vi "idontcare2.vi"() -> ()   [LabVIEW 2013]
panel:
  out "2D Picture":picture
  in  "Send Button":bool
  in  "GAIN2":dbl
  in  "GAIN1":dbl
  out "Rec Extra 4 Angle":dbl=2.8
  out "Rec Extra 3 Velocity":dbl=2.9
  out "Y":dbl=11.0
  out "X":dbl=3.0
  in  "Size of Rectangle":dbl=25.0
  in  "Display History":bool=TRUE
  in  "stop":bool
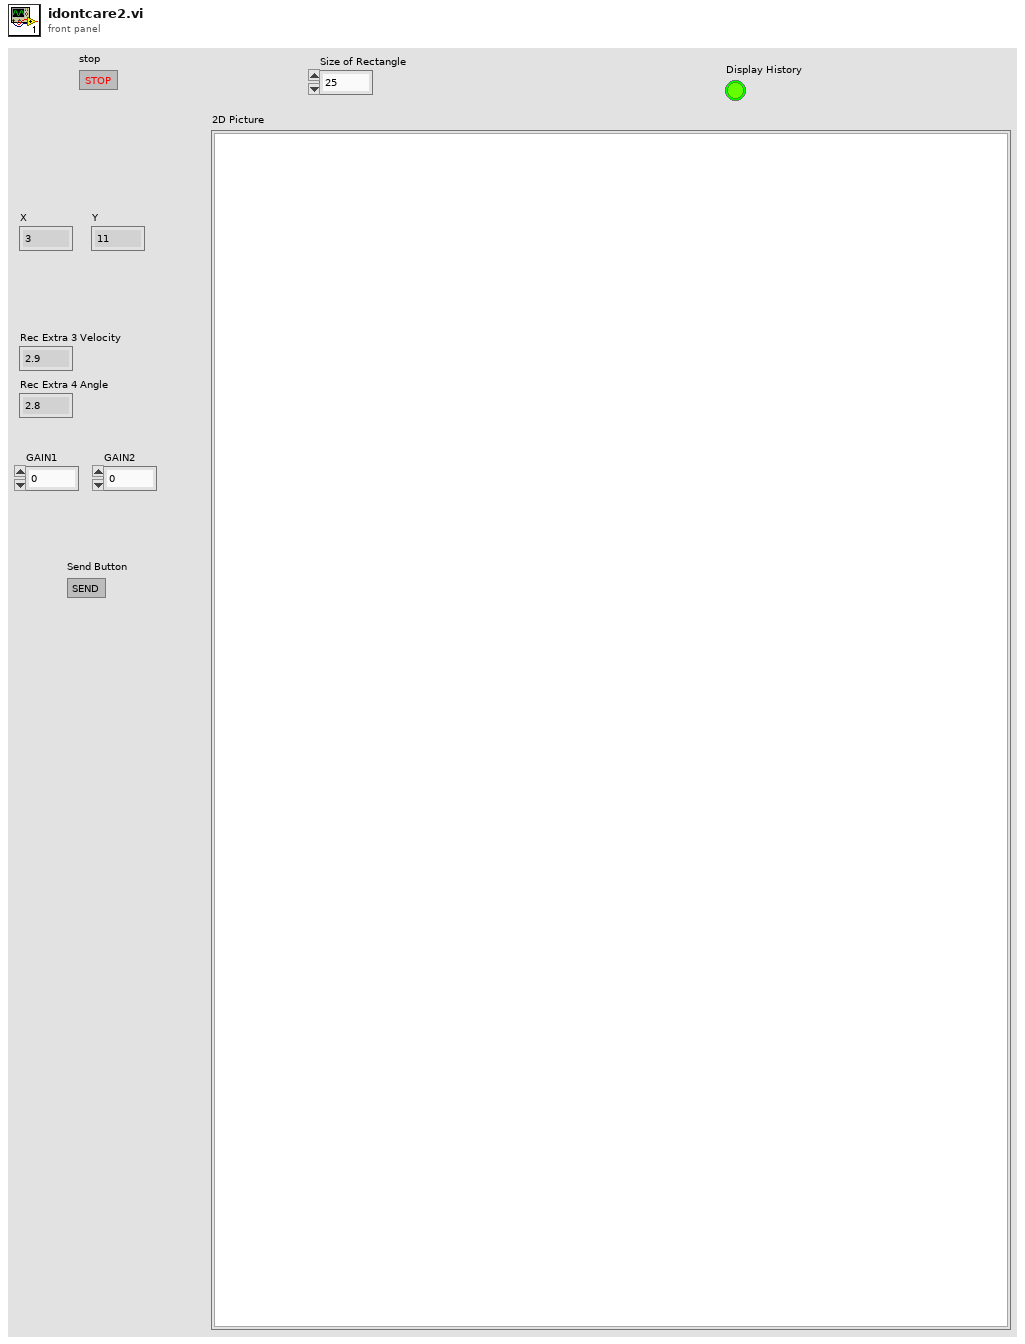
[diagram p1: front panel]
types:
  T1 = cluster{"Width":u16, "Style":enum32{"Solid", "Dash", "Dot", "DashDot", "DashDotDot"}}
  T2 = enum16{"Standard", "Buffered", "CRLF", "Immediate"}
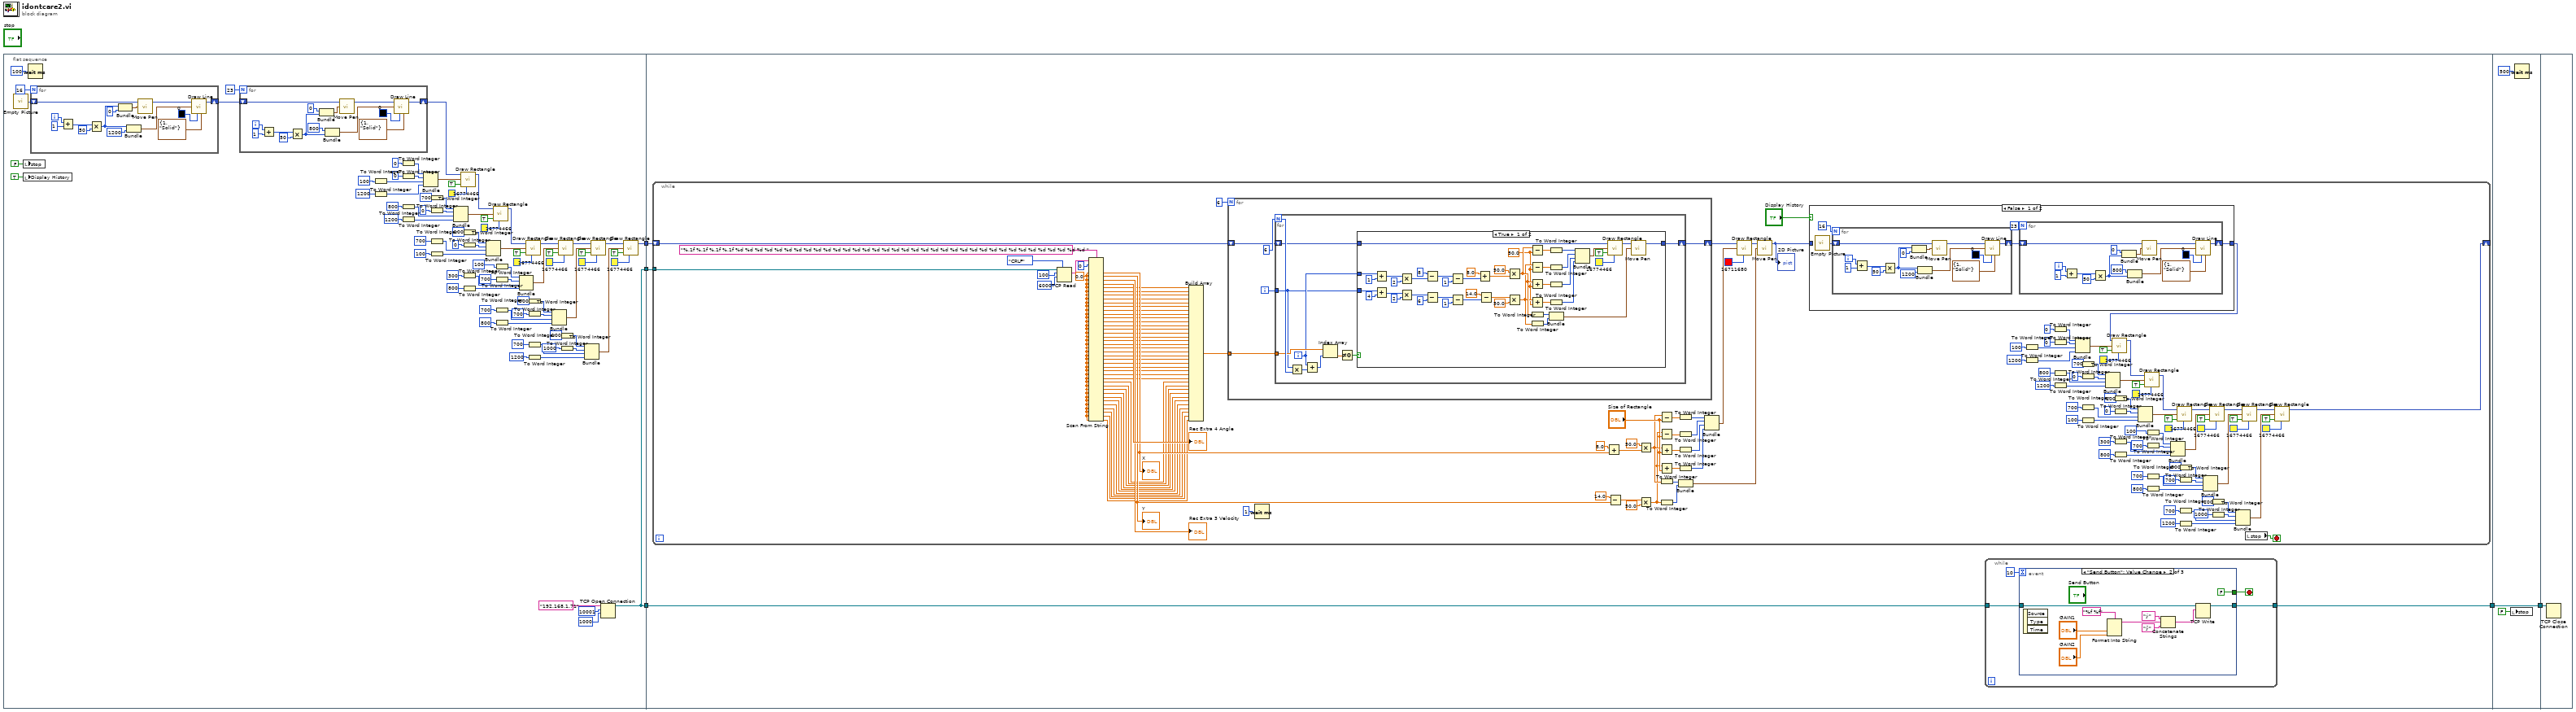
[diagram p0: block diagram]
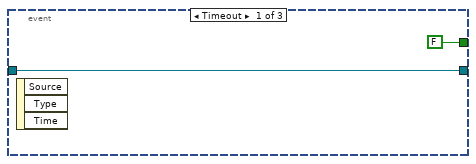
[diagram p4: hidden frame]
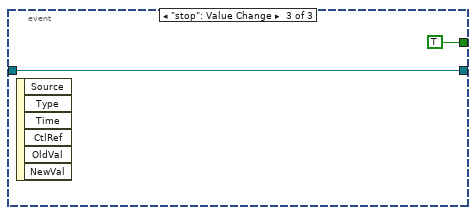
[diagram p5: hidden frame]
diagram:
  n1 = flat-sequence {
    tunnel: [w6] -> w5
    tunnel: [w83] -> w4
    tunnel: [w83] -> w3
    tunnel: w5 -> [w121]
    tunnel: w4 -> [w120]
    tunnel: w3 -> [w119]
    tunnel: [w118] -> w1
    tunnel: [w386] -> w2
    tunnel: w1 -> [w386]
    tunnel: w2 -> [w389]
    frame #0 {
      n2 = call "Empty Picture"() -> ("empty picture"=w82:picture)
      n3 = local write "stop"(FALSE) -> ()
      n4 = local write "Display History"(TRUE) -> ()
      n5 = Wait (ms)(milliseconds to wait=u32 100) -> ()  [unwired: 1 out]
      n6 = for {
        N: 16 -> [_]
        shift-right: [w106] -> w80
        shift-left: w82 -> [w117]
        i -> [w113]
        n7 = Add(x=w113, y=1) -> (x+y=w115:i32)
        n8 = Multiply(x=w115, y=50) -> (x*y=w109:i32)
        n9 = Bundle(w109, 0) -> (w111:cluster{i32, i32})  [unwired: 1 in]
        n10 = Bundle(w109, 1200) -> (w107:cluster{i32, i32})  [unwired: 1 in]
        n11 = call <vilib>:"Move Pen.vi"("new position"=w111, "picture"=w117) -> ("new picture"=w110:picture)  [unwired: 3 in]
        n12 = call <vilib>:"Draw Line.vi"("picture"=w110, "end point"=w107, "color(black)"=u32 0, "pen"=T1 {"Width"=1, "Style"=enum."Solid"}) -> ("new picture"=w106:picture)  [unwired: 5 in]
      }
      n13 = for {
        N: 23 -> [_]
        shift-right: [w95] -> w67
        shift-left: w80 -> [w103]
        i -> [w99]
        n14 = Add(x=w99, y=1) -> (x+y=w101:i32)
        n15 = Multiply(x=w101, y=50) -> (x*y=w90:i32)
        n16 = Bundle(0, w90) -> (w98:cluster{i32, i32})  [unwired: 1 in]
        n17 = Bundle(800, w90) -> (w96:cluster{i32, i32})  [unwired: 1 in]
        n18 = call <vilib>:"Move Pen.vi"("new position"=w98, "picture"=w103) -> ("new picture"=w97:picture)  [unwired: 3 in]
        n19 = call <vilib>:"Draw Line.vi"("picture"=w97, "end point"=w96, "color(black)"=u32 0, "pen"=T1 {"Width"=1, "Style"=enum."Solid"}) -> ("new picture"=w95:picture)  [unwired: 5 in]
      }
      n20 = To Word Integer(number=i16 100) -> (16bit integer=w76:i16)
      n21 = To Word Integer(number=i16 1200) -> (16bit integer=w75:i16)
      n22 = To Word Integer(number=0) -> (16bit integer=w78:i16)
      n23 = To Word Integer(number=i16 0) -> (16bit integer=w77:i16)
      n24 = To Word Integer(number=i16 800) -> (16bit integer=w64:i16)
      n25 = To Word Integer(number=i16 1200) -> (16bit integer=w63:i16)
      n26 = Bundle(w78, w77, w76, w75) -> (w74:cluster{i16, i16, i16, i16})  [unwired: 1 in]
      n27 = To Word Integer(number=700) -> (16bit integer=w66:i16)
      n28 = To Word Integer(number=i16 0) -> (16bit integer=w65:i16)
      n29 = To Word Integer(number=i16 700) -> (16bit integer=w53:i16)
      n30 = To Word Integer(number=i16 100) -> (16bit integer=w52:i16)
      n31 = Bundle(w66, w65, w64, w63) -> (w62:cluster{i16, i16, i16, i16})  [unwired: 1 in]
      n32 = call <vilib>:"Draw Rectangle.vi"("picture"=w67, "rect"=w74, "fill?(F)"=TRUE, "color(black)"=u32 16774466) -> ("new picture"=w11:picture)  [unwired: 5 in]
      n33 = To Word Integer(number=100) -> (16bit integer=w55:i16)
      n34 = To Word Integer(number=i16 0) -> (16bit integer=w54:i16)
      n35 = To Word Integer(number=i16 300) -> (16bit integer=w42:i16)
      n36 = To Word Integer(number=i16 800) -> (16bit integer=w41:i16)
      n37 = Bundle(w55, w54, w53, w52) -> (w51:cluster{i16, i16, i16, i16})  [unwired: 1 in]
      n38 = call <vilib>:"Draw Rectangle.vi"("picture"=w11, "rect"=w62, "fill?(F)"=TRUE, "color(black)"=u32 16774466) -> ("new picture"=w10:picture)  [unwired: 5 in]
      n39 = To Word Integer(number=100) -> (16bit integer=w44:i16)
      n40 = To Word Integer(number=i16 700) -> (16bit integer=w43:i16)
      n41 = To Word Integer(number=i16 700) -> (16bit integer=w31:i16)
      n42 = To Word Integer(number=i16 800) -> (16bit integer=w30:i16)
      n43 = Bundle(w44, w43, w42, w41) -> (w40:cluster{i16, i16, i16, i16})  [unwired: 1 in]
      n44 = call <vilib>:"Draw Rectangle.vi"("picture"=w10, "rect"=w51, "fill?(F)"=TRUE, "color(black)"=u32 16774466) -> ("new picture"=w9:picture)  [unwired: 5 in]
      n45 = To Word Integer(number=500) -> (16bit integer=w33:i16)
      n46 = To Word Integer(number=i16 700) -> (16bit integer=w32:i16)
      n47 = To Word Integer(number=i16 700) -> (16bit integer=w20:i16)
      n48 = To Word Integer(number=i16 1200) -> (16bit integer=w19:i16)
      n49 = Bundle(w33, w32, w31, w30) -> (w29:cluster{i16, i16, i16, i16})  [unwired: 1 in]
      n50 = call <vilib>:"Draw Rectangle.vi"("picture"=w9, "rect"=w40, "fill?(F)"=TRUE, "color(black)"=u32 16774466) -> ("new picture"=w8:picture)  [unwired: 5 in]
      n51 = To Word Integer(number=100) -> (16bit integer=w22:i16)
      n52 = To Word Integer(number=i16 1000) -> (16bit integer=w21:i16)
      n53 = Bundle(w22, w21, w20, w19) -> (w18:cluster{i16, i16, i16, i16})  [unwired: 1 in]
      n54 = call <vilib>:"Draw Rectangle.vi"("picture"=w8, "rect"=w29, "fill?(F)"=TRUE, "color(black)"=u32 16774466) -> ("new picture"=w7:picture)  [unwired: 5 in]
      n55 = TCP Open Connection(address="192.168.1.71", remote port or service name=u16 10001, timeout ms (60000)=1000) -> (connection ID=w83:refnum<k5>)  [unwired: 2 in, 1 out]
      n56 = call <vilib>:"Draw Rectangle.vi"("picture"=w7, "rect"=w18, "fill?(F)"=TRUE, "color(black)"=u32 16774466) -> ("new picture"=w6:picture)  [unwired: 5 in]
    }
    frame #1 {
      n57 = while {
        shift-right: [w122] -> _
        shift-left: w121 -> [w196]
        tunnel: w119 -> [w251]
        stop <- w252 stop-if-true
        w195 = 0.0 ("default value 1")
        n58 = TCP Read(connection ID=w251, bytes to read=100, 7:T2."CRLF" ("mode (standard)"), 9:6000 ("timeout ms (25000)")) -> (data out=w250:string)  [unwired: 1 in, 2 out]
        n59 = Scan From String(format string="%.1f %.1f %.1f %.1f %d %d %d %d %d %d %d %d %d %d %d %d %d %d %d %d %d %d %d %d %d %d %d %d %d %d %d %d %d %d %d %d %d %d %d %d ", input string=w250, initial scan location=u32 0, default 1=w195, default 2=w195, default 3=w195, default 4=w195, default 5=w195, default 6=w195, default 7=w195, default 8=w195, default 9=w195, default 10=w195, default 11=w195, default 12=w195, default 13=w195, default 14=w195, default 15=w195, default 16=w195, default 17=w195, default 18=w195, default 19=w195, default 20=w195, default 21=w195, default 22=w195, default 23=w195, default 24=w195, default 25=w195, default 26=w195, default 27=w195, default 28=w195, default 29=w195, default 30=w195, default 31=w195, default 32=w195, default 33=w195, default 34=w195, default 35=w195, default 36=w195, default 37=w195, default 38=w195, default 39=w195, default 40=w195) -> (output 1=w239:dbl, output 2=w237:dbl, output 3=→"Rec Extra 3 Velocity":dbl, output 4=→"Rec Extra 4 Angle":dbl, output 5=w235:dbl, output 6=w234:dbl, output 7=w233:dbl, output 8=w232:dbl, output 9=w231:dbl, output 10=w230:dbl, output 11=w229:dbl, output 12=w228:dbl, output 13=w227:dbl, output 14=w226:dbl, output 15=w225:dbl, output 16=w224:dbl, output 17=w223:dbl, output 18=w222:dbl, output 19=w221:dbl, output 20=w220:dbl, output 21=w219:dbl, output 22=w218:dbl, output 23=w217:dbl, output 24=w216:dbl, output 25=w215:dbl, output 26=w214:dbl, output 27=w213:dbl, output 28=w212:dbl, output 29=w211:dbl, output 30=w210:dbl, output 31=w209:dbl, output 32=w208:dbl, output 33=w207:dbl, output 34=w206:dbl, output 35=w205:dbl, output 36=w204:dbl, output 37=w203:dbl, output 38=w202:dbl, output 39=w201:dbl, output 40=w200:dbl)  [unwired: 1 in, 3 out]
        "X" <- w239
        "Y" <- w237
        n60 = Build Array(w235, w234, w233, w232, w231, w230, w229, w228, w227, w226, w225, w224, w223, w222, w221, w220, w219, w218, w217, w216, w215, w214, w213, w212, w211, w210, w209, w208, w207, w206, w205, w204, w203, w202, w201, w200) -> (w198:dbl[])
        n61 = for {
          N: 6 -> [_]
          tunnel: w198 -> [w276]
          shift-right: [w275] -> w197
          shift-left: w196 -> [w274]
          i -> [w277]
          n62 = for {
            N: 6 -> [w288]
            tunnel: w277 -> [w281]
            tunnel: w276 -> [w285]
            shift-right: [w280] -> w275
            shift-left: w274 -> [w279]
            i -> [w282]
            n63 = Multiply(x=w281, y=w288) -> (x*y=w287:i32)
            n64 = Add(x=w282, y=w287) -> (x+y=w286:i32)
            n65 = Index Array(array=w285, index=w286) -> (element=w284:dbl)
            n66 = Not Equal To 0?(x=w284) -> (x != 0?=w283:bool)
            n67 = case shown="True" w283 {
              tunnel: w279 -> [w298 w333]
              tunnel: w282 -> [w292 _]
              tunnel: w281 -> [w295 _]
              tunnel: [w296 w333] -> w280
              frame True {
                w302 = 50.0 ("y")
                n68 = Add(x=w292, y=1) -> (x+y=w291:i32)
                n69 = Add(x=w295, y=4) -> (x+y=w294:i32)
                n70 = Multiply(x=w291, y=2) -> (x*y=w331:i32)
                n71 = Multiply(x=w294, y=2) -> (x*y=w324:i32)
                n72 = Subtract(x=8, y=w331) -> (x-y=w329:i32)
                n73 = Subtract(x=w324, y=6) -> (x-y=w326:i32)
                n74 = Subtract(x=w329, y=1) -> (x-y=w301:i32)
                n75 = Subtract(x=w326, y=1) -> (x-y=w300:i32)
                n76 = Add(x=8.0, y=w301) -> (x+y=w308:dbl)
                n77 = Subtract(x=14.0, y=w300) -> (x-y=w303:dbl)
                n78 = Multiply(x=50.0, y=w308) -> (x*y=w307:dbl)
                n79 = Multiply(x=w303, y=50.0) -> (x*y=w306:dbl)
                n80 = Subtract(x=w307, y=w302) -> (x-y=w320:dbl)
                n81 = Subtract(x=w306, y=w302) -> (x-y=w319:dbl)
                n82 = Add(x=w307, y=w302) -> (x+y=w318:dbl)
                n83 = Add(x=w306, y=w302) -> (x+y=w317:dbl)
                n84 = To Word Integer(number=w307) -> (16bit integer=w310:i16)
                n85 = To Word Integer(number=w306) -> (16bit integer=w309:i16)
                n86 = To Word Integer(number=w320) -> (16bit integer=w316:i16)
                n87 = To Word Integer(number=w319) -> (16bit integer=w315:i16)
                n88 = To Word Integer(number=w318) -> (16bit integer=w314:i16)
                n89 = To Word Integer(number=w317) -> (16bit integer=w313:i16)
                n90 = Bundle(w310, w309) -> (w297:cluster{i16, i16})  [unwired: 1 in]
                n91 = Bundle(w316, w315, w314, w313) -> (w312:cluster{i16, i16, i16, i16})  [unwired: 1 in]
                n92 = call <vilib>:"Draw Rectangle.vi"("picture"=w298, "rect"=w312, "fill?(F)"=TRUE, "color(black)"=u32 16774466) -> ("new picture"=w299:picture)  [unwired: 5 in]
                n93 = call <vilib>:"Move Pen.vi"("new position"=w297, "picture"=w299) -> ("new picture"=w296:picture)  [unwired: 3 in]
              }
              frame False {
              }
            }
          }
        }
        n94 = Wait (ms)(milliseconds to wait=u32 1) -> ()  [unwired: 1 out]
        n95 = Add(x=8.0, y=w239) -> (x+y=w246:dbl)
        n96 = Subtract(x=14.0, y=w237) -> (x-y=w236:dbl)
        n97 = Multiply(x=50.0, y=w246) -> (x*y=w244:dbl)
        n98 = Multiply(x=w236, y=50.0) -> (x*y=w243:dbl)
        n99 = Subtract(x=w244, y="Size of Rectangle") -> (x-y=w263:dbl)
        n100 = Subtract(x=w243, y="Size of Rectangle") -> (x-y=w262:dbl)
        n101 = Add(x=w244, y="Size of Rectangle") -> (x+y=w261:dbl)
        n102 = Add(x=w243, y="Size of Rectangle") -> (x+y=w260:dbl)
        n103 = To Word Integer(number=w244) -> (16bit integer=w248:i16)
        n104 = To Word Integer(number=w243) -> (16bit integer=w247:i16)
        n105 = To Word Integer(number=w263) -> (16bit integer=w259:i16)
        n106 = To Word Integer(number=w262) -> (16bit integer=w258:i16)
        n107 = To Word Integer(number=w261) -> (16bit integer=w257:i16)
        n108 = To Word Integer(number=w260) -> (16bit integer=w256:i16)
        n109 = Bundle(w248, w247) -> (w249:cluster{i16, i16})  [unwired: 1 in]
        n110 = Bundle(w259, w258, w257, w256) -> (w255:cluster{i16, i16, i16, i16})  [unwired: 1 in]
        n111 = call <vilib>:"Draw Rectangle.vi"("picture"=w197, "rect"=w255, "color(black)"=u32 16711680) -> ("new picture"=w245:picture)  [unwired: 6 in]
        n112 = call <vilib>:"Move Pen.vi"("new position"=w249, "picture"=w245) -> ("new picture"=w241:picture)  [unwired: 3 in]
        "2D Picture" <- w241
        n113 = case shown="False" "Display History" {
          tunnel: [w335 w367] -> w123
          tunnel: w241 -> [_ w367]
          frame False {
            n114 = call "Empty Picture"() -> ("empty picture"=w338:picture)
            n115 = for {
              N: 16 -> [_]
              shift-right: [w355] -> w336
              shift-left: w338 -> [w366]
              i -> [w362]
              n116 = Add(x=w362, y=1) -> (x+y=w364:i32)
              n117 = Multiply(x=w364, y=50) -> (x*y=w358:i32)
              n118 = Bundle(w358, 0) -> (w360:cluster{i32, i32})  [unwired: 1 in]
              n119 = Bundle(w358, 1200) -> (w356:cluster{i32, i32})  [unwired: 1 in]
              n120 = call <vilib>:"Move Pen.vi"("new position"=w360, "picture"=w366) -> ("new picture"=w359:picture)  [unwired: 3 in]
              n121 = call <vilib>:"Draw Line.vi"("picture"=w359, "end point"=w356, "color(black)"=u32 0, "pen"=T1 {"Width"=1, "Style"=enum."Solid"}) -> ("new picture"=w355:picture)  [unwired: 5 in]
            }
            n122 = for {
              N: 23 -> [_]
              shift-right: [w344] -> w335
              shift-left: w336 -> [w352]
              i -> [w348]
              n123 = Add(x=w348, y=1) -> (x+y=w350:i32)
              n124 = Multiply(x=w350, y=50) -> (x*y=w339:i32)
              n125 = Bundle(0, w339) -> (w347:cluster{i32, i32})  [unwired: 1 in]
              n126 = Bundle(800, w339) -> (w345:cluster{i32, i32})  [unwired: 1 in]
              n127 = call <vilib>:"Move Pen.vi"("new position"=w347, "picture"=w352) -> ("new picture"=w346:picture)  [unwired: 3 in]
              n128 = call <vilib>:"Draw Line.vi"("picture"=w346, "end point"=w345, "color(black)"=u32 0, "pen"=T1 {"Width"=1, "Style"=enum."Solid"}) -> ("new picture"=w344:picture)  [unwired: 5 in]
            }
          }
          frame True {
          }
        }
        n129 = To Word Integer(number=i16 100) -> (16bit integer=w192:i16)
        n130 = To Word Integer(number=i16 1200) -> (16bit integer=w191:i16)
        n131 = To Word Integer(number=0) -> (16bit integer=w194:i16)
        n132 = To Word Integer(number=i16 0) -> (16bit integer=w193:i16)
        n133 = To Word Integer(number=i16 800) -> (16bit integer=w181:i16)
        n134 = To Word Integer(number=i16 1200) -> (16bit integer=w180:i16)
        n135 = Bundle(w194, w193, w192, w191) -> (w190:cluster{i16, i16, i16, i16})  [unwired: 1 in]
        n136 = To Word Integer(number=700) -> (16bit integer=w183:i16)
        n137 = To Word Integer(number=i16 0) -> (16bit integer=w182:i16)
        n138 = To Word Integer(number=i16 700) -> (16bit integer=w170:i16)
        n139 = To Word Integer(number=i16 100) -> (16bit integer=w169:i16)
        n140 = Bundle(w183, w182, w181, w180) -> (w179:cluster{i16, i16, i16, i16})  [unwired: 1 in]
        n141 = call <vilib>:"Draw Rectangle.vi"("picture"=w123, "rect"=w190, "fill?(F)"=TRUE, "color(black)"=u32 16774466) -> ("new picture"=w128:picture)  [unwired: 5 in]
        n142 = To Word Integer(number=100) -> (16bit integer=w172:i16)
        n143 = To Word Integer(number=i16 0) -> (16bit integer=w171:i16)
        n144 = To Word Integer(number=i16 300) -> (16bit integer=w159:i16)
        n145 = To Word Integer(number=i16 800) -> (16bit integer=w158:i16)
        n146 = Bundle(w172, w171, w170, w169) -> (w168:cluster{i16, i16, i16, i16})  [unwired: 1 in]
        n147 = call <vilib>:"Draw Rectangle.vi"("picture"=w128, "rect"=w179, "fill?(F)"=TRUE, "color(black)"=u32 16774466) -> ("new picture"=w127:picture)  [unwired: 5 in]
        n148 = To Word Integer(number=100) -> (16bit integer=w161:i16)
        n149 = To Word Integer(number=i16 700) -> (16bit integer=w160:i16)
        n150 = To Word Integer(number=i16 700) -> (16bit integer=w148:i16)
        n151 = To Word Integer(number=i16 800) -> (16bit integer=w147:i16)
        n152 = Bundle(w161, w160, w159, w158) -> (w157:cluster{i16, i16, i16, i16})  [unwired: 1 in]
        n153 = call <vilib>:"Draw Rectangle.vi"("picture"=w127, "rect"=w168, "fill?(F)"=TRUE, "color(black)"=u32 16774466) -> ("new picture"=w126:picture)  [unwired: 5 in]
        n154 = To Word Integer(number=500) -> (16bit integer=w150:i16)
        n155 = To Word Integer(number=i16 700) -> (16bit integer=w149:i16)
        n156 = To Word Integer(number=i16 700) -> (16bit integer=w137:i16)
        n157 = To Word Integer(number=i16 1200) -> (16bit integer=w136:i16)
        n158 = Bundle(w150, w149, w148, w147) -> (w146:cluster{i16, i16, i16, i16})  [unwired: 1 in]
        n159 = call <vilib>:"Draw Rectangle.vi"("picture"=w126, "rect"=w157, "fill?(F)"=TRUE, "color(black)"=u32 16774466) -> ("new picture"=w125:picture)  [unwired: 5 in]
        n160 = To Word Integer(number=100) -> (16bit integer=w139:i16)
        n161 = To Word Integer(number=i16 1000) -> (16bit integer=w138:i16)
        n162 = Bundle(w139, w138, w137, w136) -> (w135:cluster{i16, i16, i16, i16})  [unwired: 1 in]
        n163 = call <vilib>:"Draw Rectangle.vi"("picture"=w125, "rect"=w146, "fill?(F)"=TRUE, "color(black)"=u32 16774466) -> ("new picture"=w124:picture)  [unwired: 5 in]
        n164 = local read "stop"() -> (w252:bool)
        n165 = call <vilib>:"Draw Rectangle.vi"("picture"=w124, "rect"=w135, "fill?(F)"=TRUE, "color(black)"=u32 16774466) -> ("new picture"=w122:picture)  [unwired: 5 in]
      }
      n166 = while {
        tunnel: w120 -> [w370]
        tunnel: [w369] -> w118
        stop <- w368 stop-if-true
        n167 = event shown="[1] \"Send Button\": Value Change" {
          selector: _ -> [_ _ _]
          dyn-events: _ -> [_ _ _]
          timeout: 10 -> [_ _ _]
          tunnel: w370 -> [w373 w376 w384]
          tunnel: [w373 w375 w384] -> w369
          tunnel: [FALSE FALSE TRUE] -> w368
          event Timeout {
            n168 = event-data() -> ()  [unwired: 1 in, 3 out]
          }
          event "Send Button": Value Change {
            n169 = event-data() -> ()  [unwired: 1 in, 3 out]
            n170 = Format Into String(format string="%f %f", "GAIN1", "GAIN2") -> (resulting string=w378:string)  [unwired: 2 in, 1 out]
            n171 = Concatenate Strings("ý" ("string"), w378, "ÿ" ("string")) -> (w377:string)
            n172 = TCP Write(connection ID=w376, data in=w377) -> (connection ID out=w375:refnum<k5>)  [unwired: 2 in, 2 out]
          }
          event "stop": Value Change {
            n173 = event-data() -> ()  [unwired: 1 in, 6 out]
          }
        }
      }
    }
    frame #2 {
      n174 = local write "stop"(FALSE) -> ()
      n175 = Wait (ms)(milliseconds to wait=u32 500) -> ()  [unwired: 1 out]
    }
    frame #3 {
      n176 = TCP Close Connection(connection ID=w389) -> ()  [unwired: 2 in, 2 out]
    }
  }
